vi "Log Data.vi"(0 "Test Inputs":T2={"Load Current 1 in A"=0.0, "Load Current 2 in A"=0.0, "Duration of the pulse in Second"=0.0, "Nominal Output Voltage in V"=0.0, "Ref Voltage level for Settling Time Calc"=0.0, "% of Vnom for Settling Time Calc"=0.0, "Settling Time Calc Option"=enum."Voltage Level ", "Advance Setting"={"Prepare"={"Power Test Board.Voltage Level (V)"=0.0, "Power Test Board.Current Limit (A)"=0.0, "Sense Resistance (Ohm)"=1.0, "Fgen.Sample Rate (Sample/s)"=1.0}, "Stimulus And Measure"={"Fgen.Offset (V)"=0.0}}, "Save Transient Graph?"=FALSE, "Input Voltage in V"=0.0, "Save Scope Raw Data?"=FALSE, "Delay - t1 in s"=0.0, "Delay - t2 in s"=0.0, "Auto Scale Y-Axis?"=FALSE, "Shunt Resistance (Ohm)"=0.0, "Slew Rate (A/us)"=0.0, "Measure Rising Edge Slew Rate?"=TRUE, "Measure Falling Edge Slew Rate?"=TRUE} {"Advance Setting"."Stimulus And Measure"."Fgen.Offset (V)" min=1.0 format="%#_6p"; "Advance Setting"."Prepare"."Power Test Board.Current Limit (A)" min=1.0 format="%#_6p"; "Advance Setting"."Prepare"."Power Test Board.Voltage Level (V)" min=1.0 format="%#_6p"; "Advance Setting"."Prepare"."Fgen.Sample Rate (Sample/s)" min=1.0 format="%#_6p"; "Advance Setting"."Prepare"."Sense Resistance (Ohm)" min=1.0 format="%#_6p"; "Duration of the pulse in Second" format="%#.5g"; "Load Current 1 in A" format="%#.5g"}, 1 "Save Scope Raw Data?":bool, 5 "Test Results":T1 {"Falling Edge - Measured Slew Rate (A/us)" format="%#.5p"; "Rising Edge - Measured Slew Rate (A/us)" format="%#.5p"; "Second Edge - Settling Time in s" format="%#.5p"; "First Edge - Settling Time in s" format="%#.5p"; "Actual Sample Rate in S/s" format="%#.5g"}, 7 "DataLogger File Path":path, 11 "error in (no error)":errorcluster) -> (15 "error out":errorcluster)   [LabVIEW 2020, in "LDO Load Transient_AWG.lvlib"]
uses:
  LDO Load Transient_AWG.lvlib
  Typedefs/Test Inputs.ctl
  Typedefs/Settling Time Calc Option.ctl
  Typedefs/Advance Settings.ctl
  Typedefs/Adv Settings Setup Instr.ctl
  Typedefs/Adv Settings Stimulus and Measure.ctl
  Typedefs/Test Results.ctl
  <vilib>/Utility/file.llb/Write Delimited Spreadsheet (string).vi
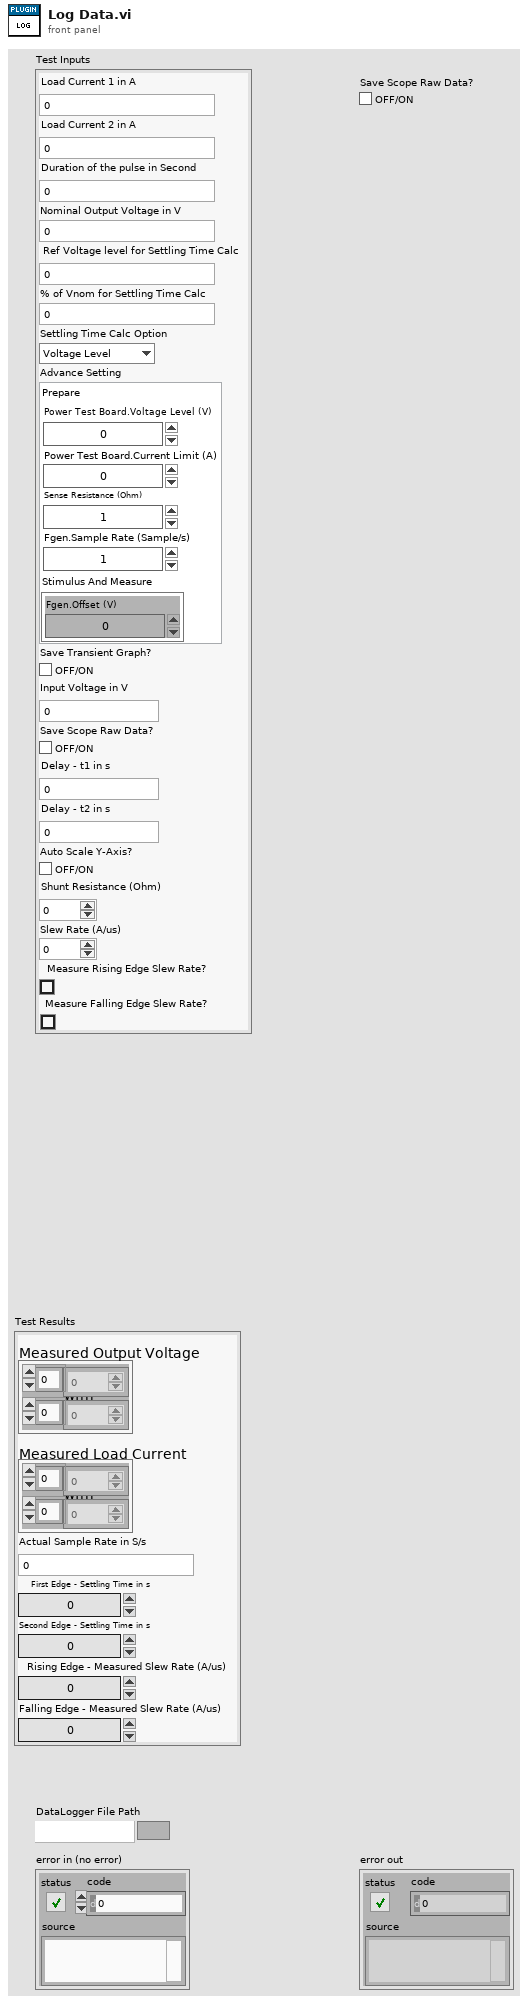
[diagram p1: front panel]
types:
  T1 = typedef "LDO Load Transient_AWG.lvlib/Test Results.ctl" = cluster{"Measured Output Voltage":cluster{"x-axis":dbl[], "wfm":dbl[]}, "Measured Load Current":cluster{"x-axis":dbl[], "wfm":dbl[]}, "Actual Sample Rate in S/s":dbl, "First Edge - Settling Time in s":dbl, "Second Edge - Settling Time in s":dbl, "Rising Edge - Measured Slew Rate (A/us)":dbl, "Falling Edge - Measured Slew Rate (A/us)":dbl}
  T2 = typedef "LDO Load Transient_AWG.lvlib/Test Inputs.ctl" = cluster{"Load Current 1 in A":dbl, "Load Current 2 in A":dbl, "Duration of the pulse in Second":dbl, "Nominal Output Voltage in V":dbl, "Ref Voltage level for Settling Time Calc":dbl, "% of Vnom for Settling Time Calc":dbl, "Settling Time Calc Option":T3, "Advance Setting":T4, "Save Transient Graph?":bool, "Input Voltage in V":dbl, "Save Scope Raw Data?":bool, "Delay - t1 in s":dbl, "Delay - t2 in s":dbl, "Auto Scale Y-Axis?":bool, "Shunt Resistance (Ohm)":dbl, "Slew Rate (A/us)":dbl, "Measure Rising Edge Slew Rate?":bool, "Measure Falling Edge Slew Rate?":bool}
  T3 = typedef "LDO Load Transient_AWG.lvlib/Settling Time Calc Option.ctl" = enum16{"Voltage Level ", "Percentage of Vnom"}
  T4 = typedef "LDO Load Transient_AWG.lvlib/Advance Settings.ctl" = cluster{"Prepare":T5, "Stimulus And Measure":T6}
  T5 = typedef "LDO Load Transient_AWG.lvlib/Adv Settings Setup Instr.ctl" = cluster{"Power Test Board.Voltage Level (V)":dbl, "Power Test Board.Current Limit (A)":dbl, "Sense Resistance (Ohm)":dbl, "Fgen.Sample Rate (Sample/s)":dbl}
  T6 = typedef "LDO Load Transient_AWG.lvlib/Adv Settings Stimulus and Measure.ctl" = cluster{"Fgen.Offset (V)":dbl}
  T7 = enum16{"open", "replace", "create", "open or create", "replace or create", "replace or create with confirmation"}
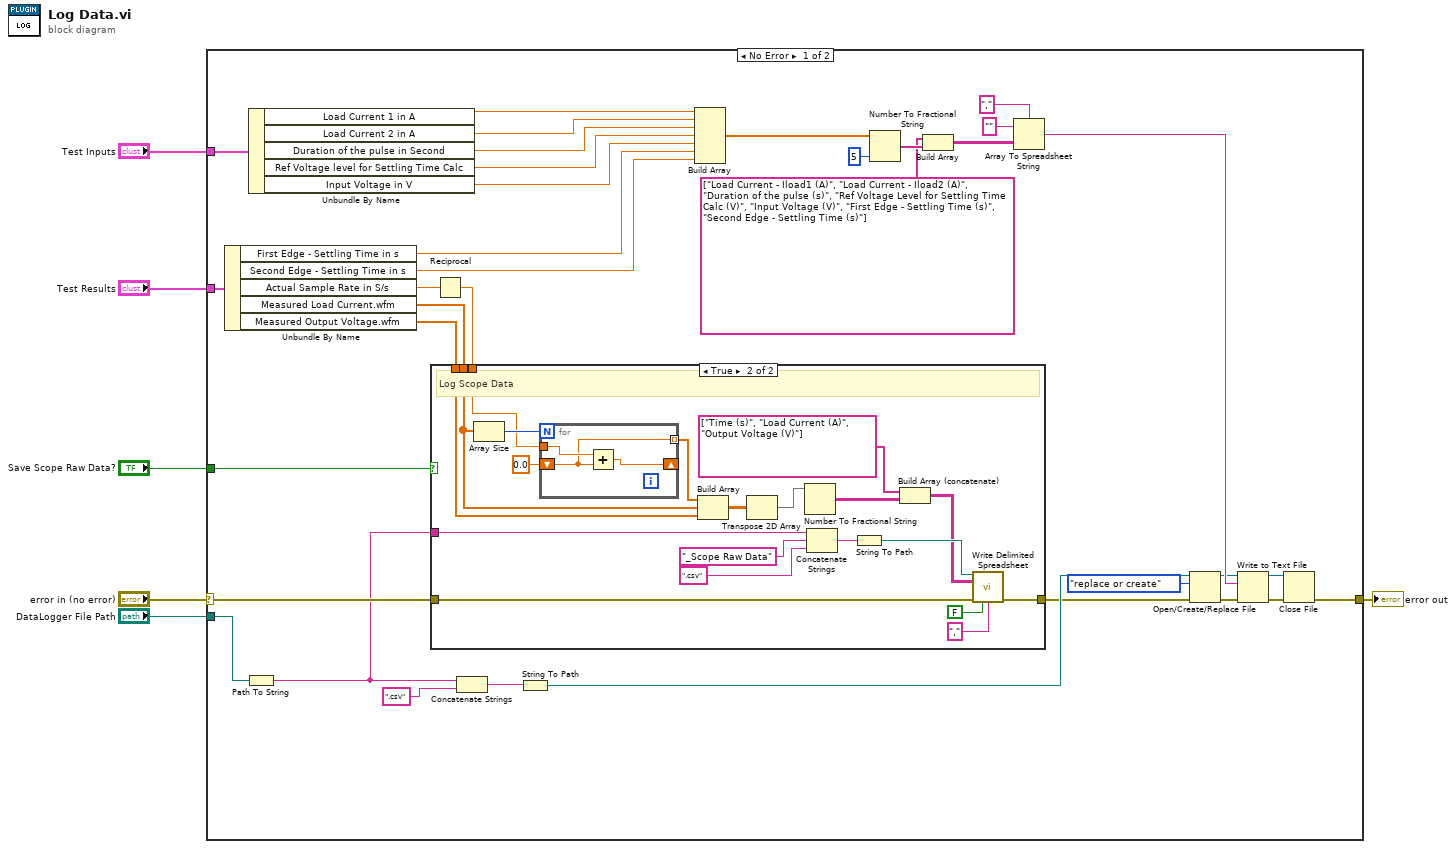
[diagram p0: block diagram]
diagram:
  n1 = case shown="No Error" "error in (no error)" {
    selector: "error in (no error)" -> [w16 w66]
    tunnel: [w38 w66] -> w5
    tunnel: "Test Inputs" -> [w41 _]
    tunnel: "Test Results" -> [w40 _]
    tunnel: "DataLogger File Path" -> [w24 _]
    tunnel: "Save Scope Raw Data?" -> [w13 _]
    frame No Error {
      n2 = Unbundle By Name(w40) -> ("First Edge - Settling Time in s"=w8:dbl, "Second Edge - Settling Time in s"=w7:dbl, "Actual Sample Rate in S/s"=w12:dbl, "Measured Load Current.wfm"=w10:dbl[], "Measured Output Voltage.wfm"=w9:dbl[])
      n3 = Path To String(path=w24) -> (string=w14:string)
      n4 = Unbundle By Name(w41) -> ("Load Current 1 in A"=w34:dbl, "Load Current 2 in A"=w39:dbl, "Duration of the pulse in Second"=w23:dbl, "Ref Voltage level for Settling Time Calc"=w21:dbl, "Input Voltage in V"=w20:dbl)
      n5 = Reciprocal(x=w12) -> (1/x=w11:dbl)
      n6 = case shown="True" w13 {
        tunnel: w16 -> [w42 w62]
        tunnel: [w42 w61] -> w15
        tunnel: w14 -> [_ w58]
        tunnel: w11 -> [_ w54]
        tunnel: w10 -> [_ w51]
        tunnel: w9 -> [_ w50]
        frame False {
          # "Skip Scope Log File"
        }
        frame True {
          # "Log Scope Data"
          n7 = Array Size(array=w51) -> (size(s)=w55:i32)
          n8 = for {
            N: w55 -> [_]
            tunnel: w54 -> [w64]
            shift-right: [w65] -> _
            shift-left: 0.0 -> [w63]
            tunnel: [w63] -> w52 mode=indexing
            n9 = Add(x=w64, y=w63) -> (x+y=w65:dbl)
          }
          n10 = Build Array(w52, w51, w50) -> (w49:dbl[][])
          n11 = Transpose 2D Array(2D array=w49) -> (transposed array=w46:dbl[][])
          n12 = Number To Fractional String(number=w46) -> (F-format string=w45:string[][])  [unwired: 3 in]
          n13 = Concatenate Strings(w58, "_Scope Raw Data" ("string"), ".csv" ("format string")) -> (w59:string)
          n14 = String To Path(string=w59) -> (path=w56:path)
          n15 = Build Array (concatenate)(string[] ["Time (s)", "Load Current (A)", "Output Voltage (V)"], w45) -> (w44:string[][])
          n16 = call-poly <vilib>:"Write Delimited Spreadsheet.vi"("file path (dialog if empty)"=w56, "2D data"=w44, "error in (no error)"=w62, "transpose? (no:F)"=FALSE, "delimiter (\\t)"="," ("delimiter (\\t)")) -> ("error out"=w61:errorcluster)  [unwired: 9 in, 1 out]
        }
      }
      n17 = Concatenate Strings(w14, ".csv" ("format string")) -> (w26:string)
      n18 = String To Path(string=w26) -> (path=w25:path)
      n19 = Build Array(w34, w39, w23, w21, w20, w8, w7) -> (w22:dbl[])
      n20 = Number To Fractional String(number=w22, precision (6)=i16 5) -> (F-format string=w19:string[])  [unwired: 2 in]
      n21 = Build Array(string[] ["Load Current - Iload1 (A)", "Load Current - Iload2 (A)", "Duration of the pulse (s)", "Ref Voltage Level for Settling Time Calc (V)", "Input Voltage (V)", "First Edge - Settling Time (s)", "Second Edge - Settling Time (s)"] ("new element/subarray"), w19) -> (w17:string[][])
      n22 = Array To Spreadsheet String(delimiter (Tab)=",", array=w17, 3:"" ("format string")) -> (spreadsheet string=w35:string)
      n23 = Open/Create/Replace File(file path (use dialog)=w25, error in=w15, operation (0:open)=T7."replace or create") -> (refnum out=w30:refnum<file>, error out=w32:errorcluster)  [unwired: 3 in, 1 out]
      n24 = Write to Text File(file (use dialog)=w30, text=w35, error in=w32) -> (refnum out=w29:refnum<file>, error out=w31:errorcluster)  [unwired: 1 in, 1 out]
      n25 = Close File(refnum=w29, error in=w31) -> (error out=w38:errorcluster)  [unwired: 1 out]
    }
    frame Error {
    }
  }
  "error out" <- w5
